vi "serialization tests.vi"() -> (0 "validation error":errorcluster, 1 "modules equal":bool, 2 "lines equal before serial test":bool, 3 "lines equal after serial test":bool, 4 "serialization error":errorcluster, 5 "channels equal":bool)   [LabVIEW 2018, in "Benchmark PID tests.lvlib"]
doc: "Tests the 'To String' and 'From String' methods of the Module's configuration class and ensures they are compatible."
uses:
  Benchmark PID tests.lvlib
  module/configuration/Benchmark PID configuration.lvclass
  module/configuration/Benchmark PID configuration.lvclass/Benchmark PID configuration.ctl
  <vilib>/NI/Tag Bus Module Framework/channel/TBM channel.lvclass
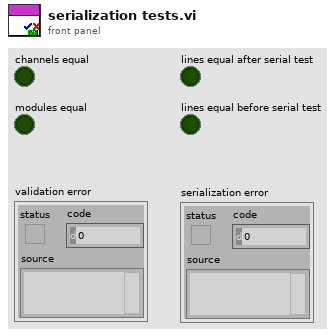
[diagram p1: front panel]
types:
  T1 = typedef "Benchmark PID configuration.lvclass/Line.ctl" = cluster{"PID Name":string, "Setpoint":refnum<class "TBM channel.lvclass">, "Variable":refnum<class "TBM channel.lvclass">, "Output":refnum<class "TBM channel.lvclass">}
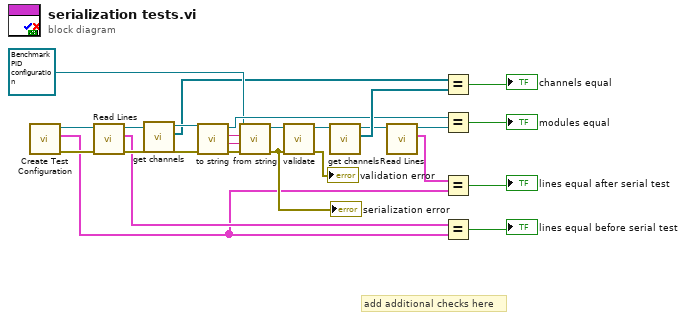
[diagram p0: block diagram]
diagram:
  # "add additional checks here"
  n1 = call "Create Test Configuration.vi"() -> ("error out"=w8:errorcluster, "Line Array"=w1:T1[], "Module Configuration"=w6:refnum<class "Benchmark PID configuration.lvclass">)  [unwired: 6 in, 3 out]
  n2 = call "Read Lines.vi"("error in (no error)"=w8, "Benchmark PID configuration in"=w6) -> ("error out"=w7:errorcluster, "Lines"=w3:T1[], "Benchmark PID configuration out"=w5:refnum<class "Benchmark PID configuration.lvclass">)  [unwired: 7 in]
  n3 = call-dynamic "get channels.vi"("Benchmark PID configuration in"=w5) -> ("channels"=w12:refnum<class "TBM channel.lvclass">[], "Benchmark PID configuration out"=w13:refnum<class "Benchmark PID configuration.lvclass">)  [unwired: 9 in]
  n4 = call-dynamic "to string.vi"("error in"=w7, "Benchmark PID configuration in"=w13) -> ("error out"=w25:errorcluster, "data"=w24:string, "version"=w23:string, "Benchmark PID configuration out"=w15:refnum<class "Benchmark PID configuration.lvclass">)  [unwired: 6 in]
  n5 = call-dynamic "from string.vi"("error in"=w25, "data"=w24, "version"=w23, "Benchmark PID configuration in"=refnum<class "Benchmark PID configuration.lvclass"> refnum ("tag bus configurable plugin module configuration")) -> ("error out"=w20:errorcluster, "Benchmark PID configuration out"=w22:refnum<class "Benchmark PID configuration.lvclass">)  [unwired: 6 in]
  "serialization error" <- w20
  n6 = call-dynamic "validate.vi"("error in"=w20, "Benchmark PID configuration in"=w22) -> ("error out"=→"validation error":errorcluster, "Benchmark PID configuration out"=w18:refnum<class "Benchmark PID configuration.lvclass">)  [unwired: 8 in]
  n7 = call-dynamic "get channels.vi"("Benchmark PID configuration in"=w18) -> ("channels"=w17:refnum<class "TBM channel.lvclass">[], "Benchmark PID configuration out"=w11:refnum<class "Benchmark PID configuration.lvclass">)  [unwired: 9 in]
  n8 = call "Read Lines.vi"("Benchmark PID configuration in"=w11) -> ("Lines"=w2:T1[], "Benchmark PID configuration out"=w10:refnum<class "Benchmark PID configuration.lvclass">)  [unwired: 8 in, 1 out]
  n9 = Equal?(x=w12, y=w17) -> (x = y?=→"channels equal":bool)
  n10 = Equal?(x=w15, y=w10) -> (x = y?=→"modules equal":bool)
  n11 = Equal?(x=w2, y=w1) -> (x = y?=→"lines equal after serial test":bool)
  n12 = Equal?(x=w3, y=w1) -> (x = y?=→"lines equal before serial test":bool)
